vi "Imaging Parameters to text array.vi"(9 "Imaging Parameters":T1[](array[typedef]), 10 "Image Ref":string[](array[string]), 11 "Image No":string[](array[string])) -> (3 "Imaging Parameters":string[][](array[string]))   [LabVIEW 2020]
uses:
  TypeDefs/Current Imaging Parameters.ctl
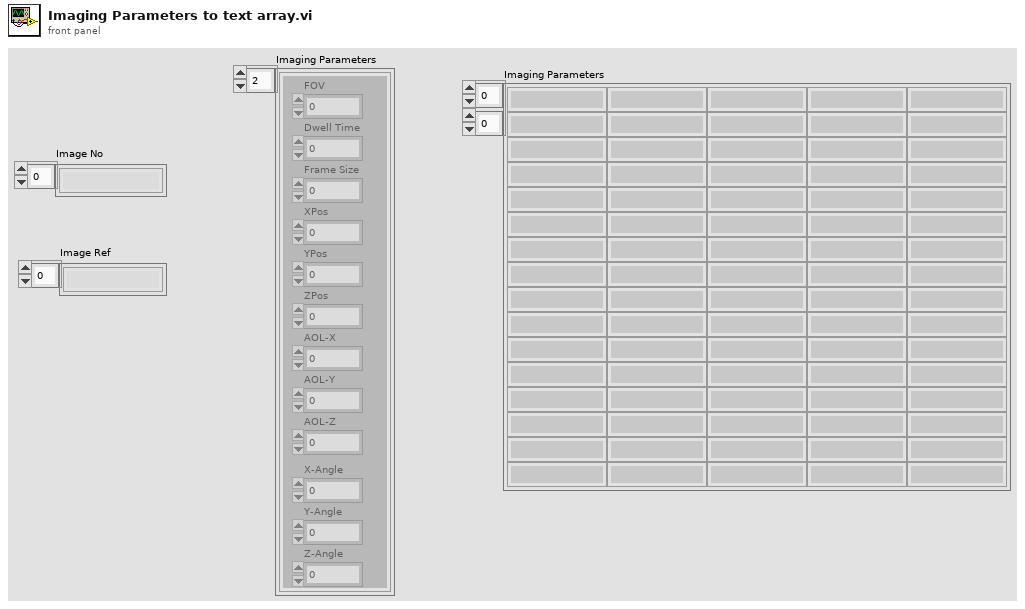
[diagram p1: front panel]
types:
  T1 = typedef "Current Imaging Parameters.ctl" = cluster{"FOV":dbl, "Dwell Time":dbl, "Frame Size":dbl, "XPos":dbl, "YPos":dbl, "ZPos":dbl, "AOL-X":dbl, "AOL-Y":dbl, "AOL-Z":dbl, "X-Angle":dbl, "Y-Angle":dbl, "Z-Angle":dbl}
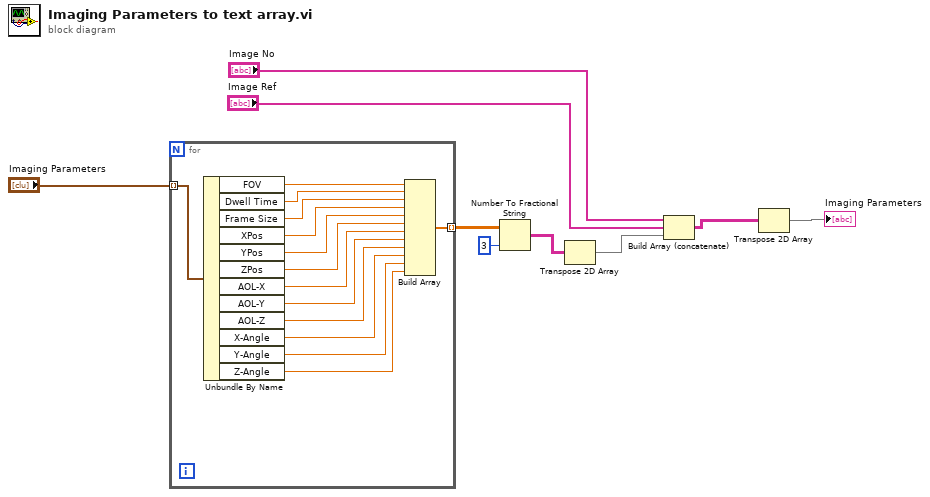
[diagram p0: block diagram]
diagram:
  n1 = for {
    tunnel: "Imaging Parameters" -> [w23] mode=indexing
    tunnel: [w10] -> w8 mode=indexing
    n2 = Unbundle By Name(w23) -> ("FOV"=w22:dbl, "Dwell Time"=w21:dbl, "Frame Size"=w20:dbl, "XPos"=w19:dbl, "YPos"=w18:dbl, "ZPos"=w17:dbl, "AOL-X"=w16:dbl, "AOL-Y"=w15:dbl, "AOL-Z"=w14:dbl, "X-Angle"=w13:dbl, "Y-Angle"=w12:dbl, "Z-Angle"=w11:dbl)
    n3 = Build Array(w22, w21, w20, w19, w18, w17, w16, w15, w14, w13, w12, w11) -> (w10:dbl[])
  }
  n4 = Number To Fractional String(number=w8, precision (6)=i16 3) -> (F-format string=w4:string[][])  [unwired: 2 in]
  n5 = Transpose 2D Array(2D array=w4) -> (transposed array=w3:string[][])
  n6 = Build Array (concatenate)("Image No", "Image Ref", w3) -> (w2:string[][])
  n7 = Transpose 2D Array(2D array=w2) -> (transposed array=→"Imaging Parameters":string[][])
